vi "fgv_system_info.vi"(7 "cmd":enum16{"read", "write"}(ring), 11 "info":cluster{"ip":string}) -> (3 "info_out":cluster{"ip":string})   [LabVIEW 2019]
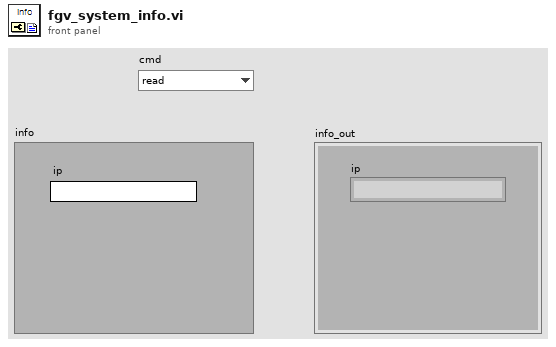
[diagram p1: front panel]
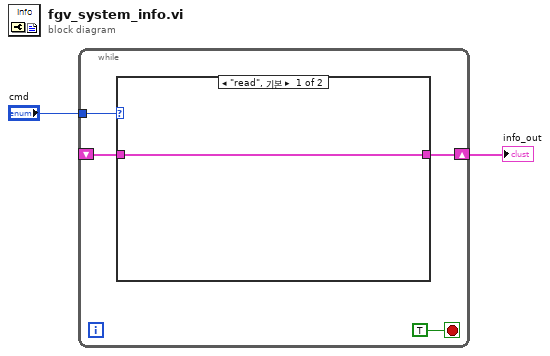
[diagram p0: block diagram]
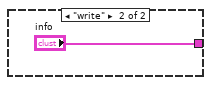
[diagram p2: hidden frame]
diagram:
  n1 = while {
    tunnel: "cmd" -> [w5]
    shift-right: [w4] -> w1
    shift-left: _ -> [w3]
    stop <- TRUE stop-if-true
    n2 = case shown="\"read\", 기본" w5 {
      tunnel: [w7 "info"] -> w4
      tunnel: w3 -> [w7 _]
      frame "read", Default {
      }
      frame "write" {
      }
    }
  }
  "info_out" <- w1
